vi "Unflatten-MouseWheelEventData.vi"(8 "error in (no error)":errorcluster, 11 "Event Binary Data":string) -> (0 "error out":errorcluster, 3 "MouseWheelEvent":T1)   [LabVIEW 2024, in "SDL3.lvlib" / "Events.lvlib"]
uses:
  Events.lvlib
  Video/WindowID--integer.ctl
  Video/Video.lvlib
  Mouse/MouseID--integer.ctl
  Mouse/Mouse.lvlib
  Mouse/MouseWheelDirection--enum.ctl
  MouseWheelEvent--cluster.ctl
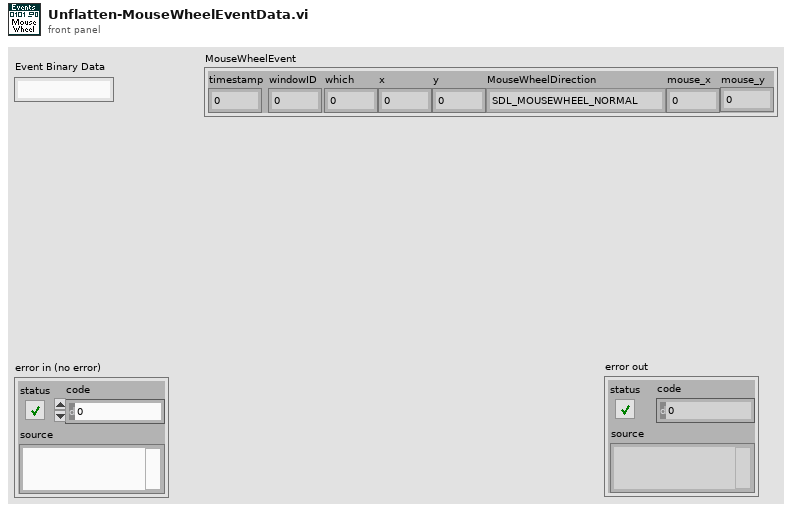
[diagram p1: front panel]
types:
  T1 = typedef "SDL3.lvlib/Events.lvlib/MouseWheelEvent--cluster.ctl" = cluster{"timestamp":u64, "windowID":T2, "which":T3, "x":sgl, "y":sgl, "MouseWheelDirection":T4, "mouse_x":sgl, "mouse_y":sgl}
  T2 = typedef "SDL3.lvlib/Video.lvlib/WindowID--integer.ctl" = u32
  T3 = typedef "SDL3.lvlib/Mouse.lvlib/MouseID--integer.ctl" = u32
  T4 = typedef "SDL3.lvlib/Mouse.lvlib/MouseWheelDirection--enum.ctl" = enum32{"SDL_MOUSEWHEEL_NORMAL", "SDL_MOUSEWHEEL_FLIPPED"}
  T5 = enum16{"big-endian, network order", "native, host order", "little-endian"}
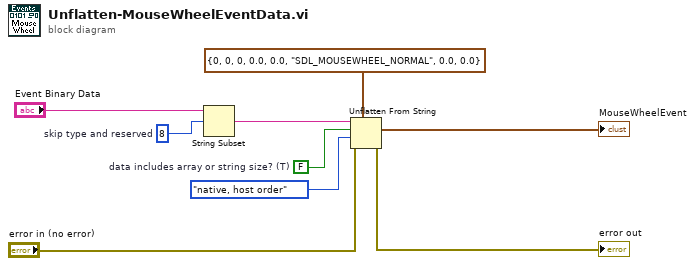
[diagram p0: block diagram]
diagram:
  w3 = 8  # skip type and reserved
  w6 = FALSE  # data includes array or string size? (T)
  n1 = String Subset(string="Event Binary Data", offset (0)=w3) -> (substring=w4:string)  [unwired: 1 in]
  n2 = Unflatten From String(type=T1 {"timestamp"=0, "windowID"=0, "which"=0, "x"=0.0, "y"=0.0, "MouseWheelDirection"=enum."SDL_MOUSEWHEEL_NORMAL", "mouse_x"=0.0, "mouse_y"=0.0} ("MouseWheelEvent"), binary string=w4, data includes array or string size? (T)=w6, byte order (0:big-endian, network order)=T5."native, host order", error in (no error)="error in (no error)") -> (value=→"MouseWheelEvent":T1, error out=→"error out":errorcluster)  [unwired: 1 out]
